vi "Open Existing Buffer.vi"(8 "error in (no error)":errorcluster, 9 "timeout (ms)":i32=2000, 11 "buffer_name":string="/example") -> (0 "error out":errorcluster, 3 "CIPC Reference":u64)   [LabVIEW 2021, in "CIF_NI_CIPC.lvlib"]
doc: "Open an existing CIPC buffer.s\n\nInputs:\n- buffer_name: name of the buffer\n- timeout: timeout in ms to wait for the CIPC buffer to be created.\n- prepend array or string size?: if true, the elements in the buffer will have their array size prepended in the data\n\nOutputs:\n- buffer_refs: reference and information on the created/opened CIPC buffer\ns"
uses:
  CIF_NI_CIPC.lvlib
  libnicipc.dll
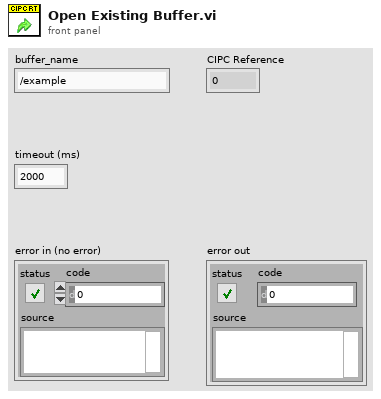
[diagram p1: front panel]
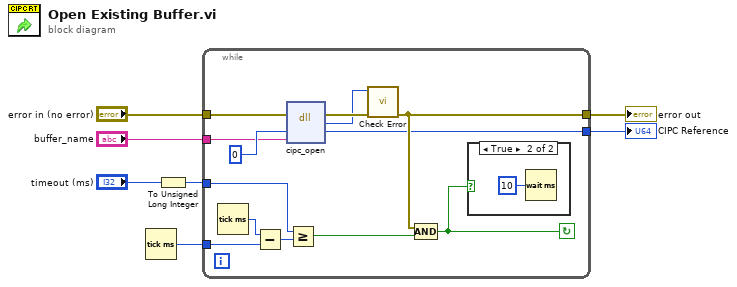
[diagram p0: block diagram]
diagram:
  n1 = Tick Count (ms)() -> (millisecond timer value=w7:u32)
  n2 = To Unsigned Long Integer(number="timeout (ms)") -> (unsigned 32bit integer=w5:u32)
  n3 = while {
    tunnel: [w11] -> w1
    tunnel: w7 -> [w16]
    tunnel: w5 -> [w14]
    tunnel: "buffer_name" -> [w12]
    tunnel: "error in (no error)" -> [w10]
    tunnel: [w9] -> w2
    stop <- w8 continue-if-true
    n4 = Tick Count (ms)() -> (millisecond timer value=w17:u32)
    n5 = Subtract(x=w17, y=w16) -> (x-y=w13:u32)
    n6 = dll-call lib="libnicipc.*" fn="cipc_open"(error in=w10, "cipc_buffer_ref"=u64 0, "name"=w12) -> (error out=w19:errorcluster, "return type"=w18:i32, "cipc_buffer_ref"=w9:u64)  [unwired: 3 in, 1 out]
    n7 = Greater Or Equal?(x=w14, y=w13) -> (x >= y?=w15:bool)
    n8 = call "Check Error.vi"("error in (no error)"=w19, "Error Code"=w18) -> ("error out"=w11:errorcluster)  [unwired: 9 in]
    n9 = Compound Arithmetic op=AND(w11, w15) -> (w8:bool)
    n10 = case shown="True" w8 {
      frame False {
      }
      frame True {
        n11 = Wait (ms)(milliseconds to wait=u32 10) -> ()  [unwired: 1 out]
      }
    }
  }
  "error out" <- w1
  "CIPC Reference" <- w2
